vi "ReadSerial.vi"(8 "error in (no error)":errorcluster, 9 "timeout (msec)":u32=200, 11 "VISA Refnum in":refnum<visa-resource-name>) -> (0 "error out":errorcluster, 2 "String Read":string="BW10\n", 3 "VISA Refnum out":refnum<visa-resource-name>)   [LabVIEW 2022 SP3]
panel:
  in  "OK Button":bool
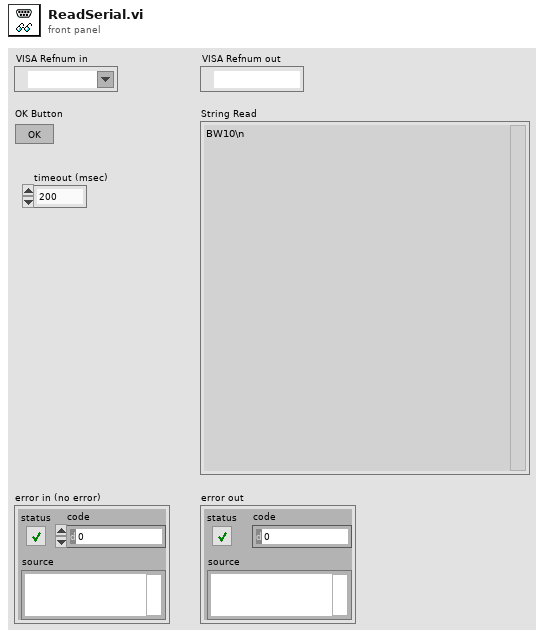
[diagram p1: front panel]
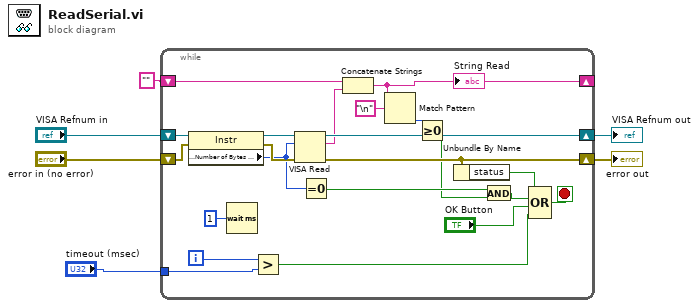
[diagram p0: block diagram]
diagram:
  n1 = while {
    shift-right: [w24] -> w3
    shift-left: "VISA Refnum in" -> [w26]
    shift-right: [w20] -> w2
    shift-left: "error in (no error)" -> [w25]
    shift-right: [w10] -> _
    shift-left: "" -> [w22]
    tunnel: "timeout (msec)" -> [w7]
    i -> [w9]
    stop <- w15 stop-if-true
    n2 = property class="Instr"(reference=w26, error in=w25) -> (reference out=w27:refnum<visa-resource-name>, error out=w28:errorcluster, "Serial Settings:Number of Bytes at Serial Port"=w17:u32)
    n3 = Wait (ms)(milliseconds to wait=u32 1) -> ()  [unwired: 1 out]
    n4 = Greater?(x=w9, y=w7) -> (0:w8:bool)
    n5 = VISA Read(VISA resource name=w27, byte count=w17, error in (no error)=w28) -> (VISA resource name out=w24:refnum<visa-resource-name>, read buffer=w21:string, error out=w20:errorcluster)  [unwired: 1 out]
    n6 = Equal To 0?(x=w17) -> (x = 0?=w16:bool)
    n7 = Concatenate Strings(w22, w21) -> (w10:string)
    "String Read" <- w10
    n8 = Match Pattern(string=w10, regular expression="\n") -> (offset past match=w11:i32)  [unwired: 1 in, 3 out]
    n9 = Greater Or Equal To 0?(x=w11) -> (x >= 0?=w14:bool)
    n10 = Unbundle By Name(w20) -> ("status"=w19:bool)
    n11 = And(x=w16, y=w14) -> (x .and. y?=w13:bool)
    n12 = Compound Arithmetic op=OR(w19, w13, "OK Button", w8) -> (w15:bool)
  }
  "VISA Refnum out" <- w3
  "error out" <- w2
